vi "Record QPDx.vi"() -> ()   [LabVIEW 2014]
uses:
  <vilib>/Analysis/3filter.llb/Savitzky-Golay Filter (DBL).vi
  <vilib>/DAQmx/create/channels.llb/DAQmx Create Channel (AI-Voltage-Basic).vi
  <vilib>/DAQmx/configure/timing.llb/DAQmx Timing (Sample Clock).vi
  <vilib>/DAQmx/read.llb/DAQmx Read (Analog 1D DBL 1Chan NSamp).vi
  <vilib>/Utility/file.llb/Write To Spreadsheet File (DBL).vi
  <vilib>/Analysis/NI_AALBase.lvlib
panel:
  in  "record time (s)":i32
  in  "intervals":i32=10
  in  "Save?":bool
  in  "Tab Control":enum32{"Raw", "Filter"}(tab)
  out "Waveform Chart":dbl[](graph)
  out "Waveform Chart 2":dbl[](graph)
  out "Histogram Graph":T1(graph)
  in  "side points":i32=6
  in  "Stop to save":bool
  in  "number of samples per channel":i32=32000
  in  "rate":dbl=32000.0 format="%0.2f"
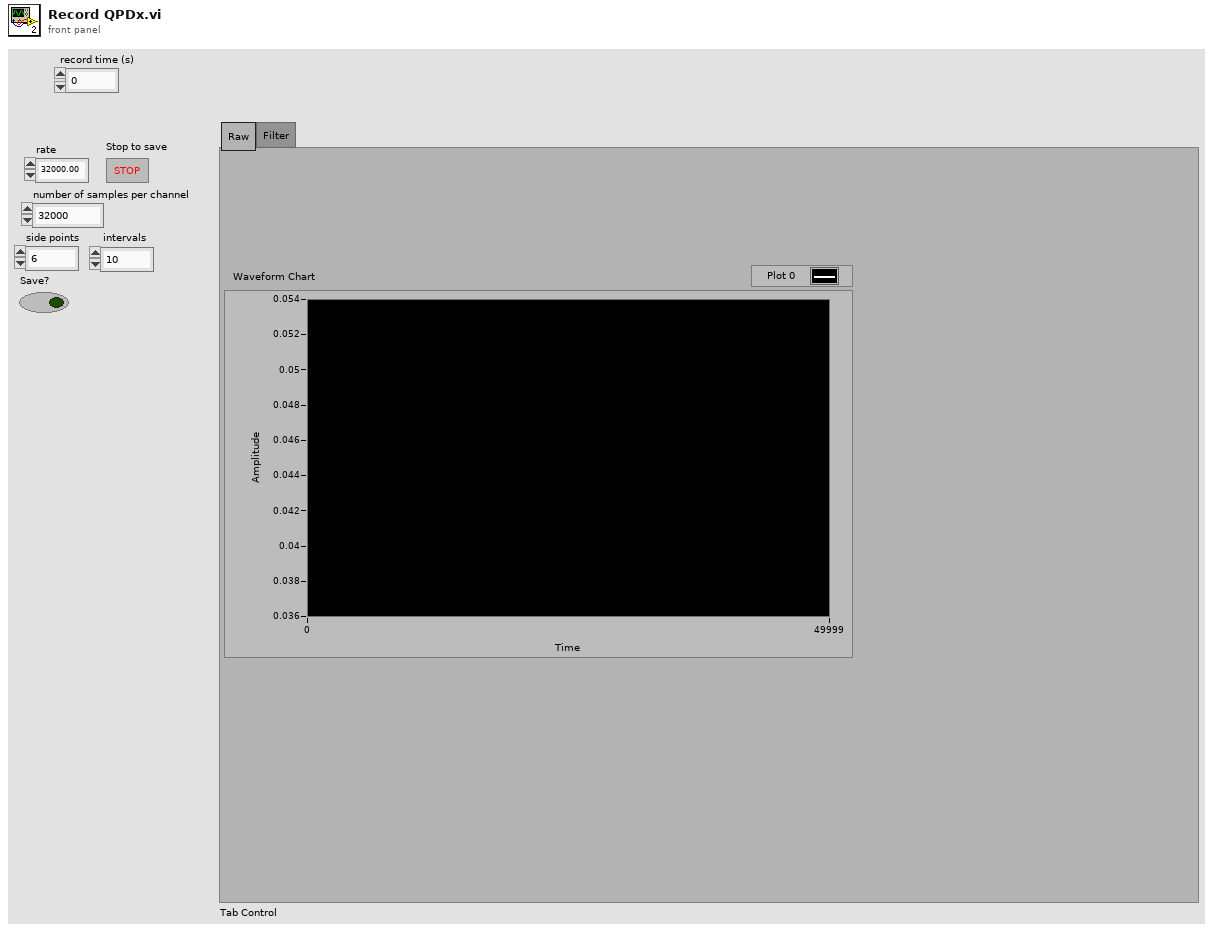
[diagram p1: front panel]
types:
  T1 = cluster{"X Values":dbl[], "Histogram: h(x)":i32[]}
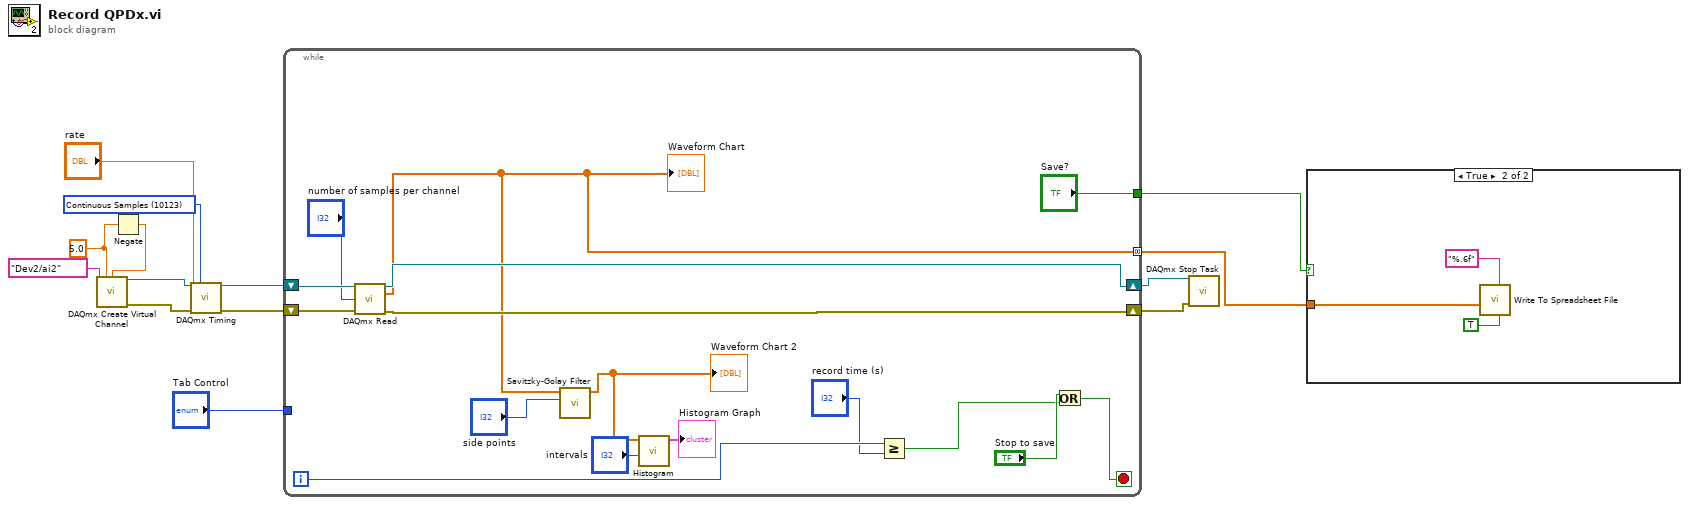
[diagram p0: block diagram]
diagram:
  w8 = 10123 items=["Finite Samples"=10178, "Continuous Samples"=10123, "Hardware Timed Single Point"=12522] ("sample mode")
  w13 = 5.0 ("maximum value")
  n1 = Negate(x=w13) -> (-x=w12:dbl)
  n2 = call-poly <vilib>:"DAQmx Create Virtual Channel.vi"("maximum value"=w13, "minimum value"=w12, "physical channels"=tag "Dev2/ai2") -> ("task out"=w10:refnum<k21>, "error out"=w11:errorcluster)  [unwired: 11 in]
  n3 = call-poly <vilib>:"DAQmx Timing.vi"("task/channels in"=w10, "sample mode"=w8, "rate"="rate", "error in"=w11) -> ("task out"=w7:refnum<k21>, "error out"=w6:errorcluster)  [unwired: 10 in]
  n4 = while {
    shift-right: [w27] -> w5
    shift-left: w7 -> [w30]
    shift-right: [w26] -> w4
    shift-left: w6 -> [w29]
    tunnel: ["Save?"] -> w3
    tunnel: [w23] -> w2 mode=concatenating
    tunnel: "Tab Control" -> [_]
    i -> [w19]
    stop <- w15 stop-if-true
    n5 = call-poly <vilib>:"DAQmx Read.vi"("task/channels in"=w30, "number of samples per channel"="number of samples per channel", "error in"=w29) -> ("task out"=w27:refnum<k21>, "data"=w23:dbl[], "error out"=w26:errorcluster)  [unwired: 10 in]
    "Waveform Chart" <- w23
    n6 = call-poly <vilib>:"Savitzky-Golay Filter.vi"("side points"="side points", "X"=w23) -> ("Filtered X"=w22:dbl[])  [unwired: 8 in, 1 out]
    "Waveform Chart 2" <- w22
    n7 = call <vilib>:"Histogram.vi"("intervals"="intervals", "X"=w22) -> ("Histogram Graph"=→"Histogram Graph":T1)  [unwired: 6 in, 3 out]
    n8 = Greater Or Equal?(x=w19, y="record time (s)") -> (x >= y?=w16:bool)
    n9 = Or(x="Stop to save", y=w16) -> (x .or. y?=w15:bool)
  }
  n10 = call <vilib>:"DAQmx Stop Task.vi"("task/channels in"=w5, "error in"=w4) -> ()  [unwired: 12 in, 2 out]
  n11 = case shown="True" w3 {
    tunnel: w2 -> [_ w33]
    frame False {
    }
    frame True {
      n12 = call-poly <vilib>:"Write To Spreadsheet File.vi"("transpose? (no:F)"=TRUE, "format (%.3f)"="%.6f", "1D data"=w33) -> ()  [unwired: 5 in, 1 out]
    }
  }
